vi "HAILO_3d_Open_Display.vi"(8 "error in (no error)":errorcluster, 10 "Rendering Type":enum16{"3D Window", "3D Off"}(ring), 11 "Camera Controller":enum16{"None", "Spherical", "Flying"}(ring)) -> (0 "error out":errorcluster, 3 "SceneWindow out":refnum<vi>)   [LabVIEW 2016]
uses:
  <vilib>/Utility/miscctls.llb/LVRectTypeDef.ctl
  <vilib>/picture/3D Picture Control/NI_3D Picture Control.lvlib
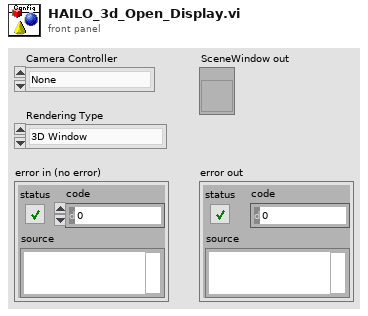
[diagram p1: front panel]
types:
  T1 = enum16{"None", "Spherical", "Flying", "Oriented"}
  T2 = enum16{"Open", "Minimized", "Maximized", "Hidden"}
  T3 = typedef "LVRectTypeDef.ctl" = cluster{"Left":i16, "Top":i16, "Right":i16, "Bottom":i16}
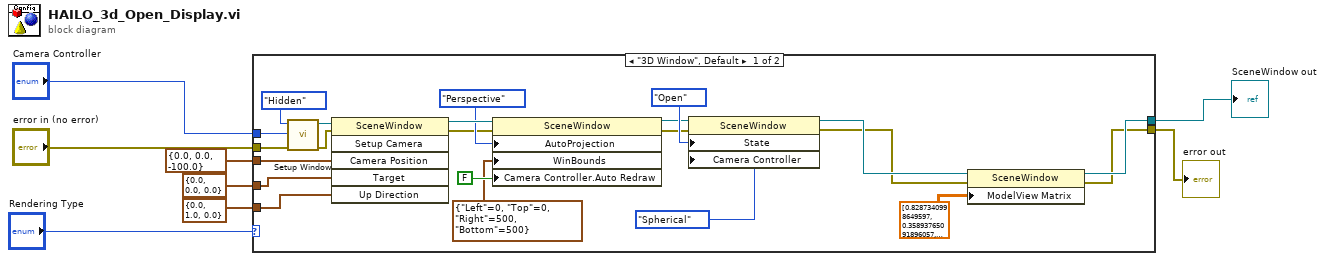
[diagram p0: block diagram]
diagram:
  n1 = case shown="\"3D Window\", Default" "Rendering Type" {
    tunnel: "Camera Controller" -> [w21 _]
    tunnel: cluster{"X":sgl, "Y":sgl, "Z":sgl} {"X"=0.0, "Y"=0.0, "Z"=-100.0} ("Camera Position") -> [w23 _]
    tunnel: cluster{"X":sgl, "Y":sgl, "Z":sgl} {"X"=0.0, "Y"=0.0, "Z"=0.0} ("Target") -> [w24 _]
    tunnel: cluster{"X":sgl, "Y":sgl, "Z":sgl} {"X"=0.0, "Y"=1.0, "Z"=0.0} ("Up Direction") -> [w25 _]
    tunnel: [w11 _] -> w6
    tunnel: [w9 w31] -> w8
    tunnel: "error in (no error)" -> [w15 w31]
    frame "3D Window", Default {
      n2 = call <vilib>:"Setup Window.vi"("error in (no error)"=w15, "Camera Controller"=w21, "Window State"=T2."Hidden") -> ("error out"=w18:errorcluster, "New Window Refnum"=w27:refnum<vi>)  [unwired: 7 out]
      n3 = invoke class="SceneWindow" method="Setup Camera"(reference=w27, error in=w18, "Camera Position"=w23, "Target"=w24, "Up Direction"=w25) -> (reference out=w26:refnum<vi>, error out=w17:errorcluster)  [unwired: 1 in, 4 out]
      n4 = property class="SceneWindow"(reference=w26, error in=w17, "AutoProjection"=enum16{"None", "Perspective", "Orthographic"}."Perspective" ("Automatic Projection Mode"), "WinBounds"=T3 {"Left"=0, "Top"=0, "Right"=500, "Bottom"=500} ("Window Bounds"), "Camera Controller.Auto Redraw"=FALSE ("Camera Controller:Auto Redraw")) -> (reference out=w19:refnum<vi>, error out=w16:errorcluster)
      n5 = property class="SceneWindow"(reference=w19, error in=w16, "State"=T2."Open" ("Window State"), "Camera Controller"=T1."Spherical" ("Camera Controller:Type")) -> (reference out=w12:refnum<vi>, error out=w10:errorcluster)
      n6 = property class="SceneWindow"(reference=w12, error in=w10, "ModelView Matrix"=sgl[][] [[0.8287341, 0.35893765, -0.42937574, 53.04154], [0.29138392, 0.3782908, 0.87863046, -7.295283], [0.47780246, -0.8532642, 0.20891382, -214.55814], [0.0, 0.0, 0.0, 1.0]]) -> (reference out=w11:refnum<vi>, error out=w9:errorcluster)
    }
    frame "3D Off" {
    }
  }
  "error out" <- w8
  "SceneWindow out" <- w6
